vi "InputProc.vi"(7 "error in":errorcluster, 8 "output cluster":T16, 9 "SensorInputData":T17, 10 "GamepadData":T18) -> (0 "error out":errorcluster, 2 "SensorInputDataOut":T17, 3 "GamepadDataOut":T18)   [LabVIEW 2014]
uses:
  Typedefs/GamepadData.ctl
  Typedefs/SensorInputData.ctl
  <vilib>/Rock Robotics/WPI/Joystick/WPI_JoystickDevRef.ctl
  <vilib>/Rock Robotics/WPI/Joystick/WPI_JoystickDeviceEnum.ctl
  <vilib>/Rock Robotics/WPI/Potentiometer/WPI_PotentiometerDevRef.ctl
  <vilib>/Rock Robotics/SystemInterfaces/Typedef/FPGA_TypedefAnalogModule.ctl
  <vilib>/Rock Robotics/SystemInterfaces/AI/FPGA_AIChannel.ctl
  <vilib>/Rock Robotics/WPI/Encoder/WPI_EncoderDevRef.ctl
  <vilib>/Rock Robotics/SystemInterfaces/Encoder/FPGA_EncoderIdx.ctl
  <vilib>/Rock Robotics/SystemInterfaces/Counter/FPGA_CounterCtrSystemIndex.ctl
  <vilib>/Rock Robotics/WPI/Encoder/WPI_EncoderType.ctl
  <vilib>/Rock Robotics/WPI/Switch/WPI_SwitchDevRef.ctl
  <vilib>/Rock Robotics/SystemInterfaces/DIO/FPGA_DIOChannel.ctl
  <vilib>/Rock Robotics/SystemInterfaces/Typedef/FPGA_TypedefDigitalModule.ctl
  <vilib>/Rock Robotics/WPI/Gyro/WPI_GyroDevRef.ctl
  <vilib>/Rock Robotics/WPI/Compressor/WPI_CompressorDevRef.ctl
  Gensubs/Bert_or_Ernie.vi
  Typedefs/JoysticksGlobal.vi
panel:
  in  "Wench Deadzone Limit":dbl=0.05 format="%#_13g"
  in  "X360 Deadzone Limit":dbl=0.3
  in  "Bert Arm Inputs":T1={"SensorMax"=0.929, "UnitMin"=-26.5, "SensorMin"=0.502, "UnitMax"=86.8}
  in  "Ernie Arm Inputs":T1={"SensorMax"=0.837, "UnitMin"=-26.7, "SensorMin"=0.444, "UnitMax"=87.4}
  out "Claw Pot Raw":dbl
  in  "Ernie StackerClamp Inputs":T1={"SensorMax"=0.852, "UnitMin"=148.3, "SensorMin"=0.477, "UnitMax"=219.6}
  in  "Ernie Stacker Inputs":T1={"SensorMax"=0.782, "UnitMin"=0.0, "SensorMin"=0.357, "UnitMax"=21.125}
  in  "Bert StackerClamp Inputs":T1={"SensorMax"=0.42, "UnitMin"=141.5, "SensorMin"=0.064, "UnitMax"=217.6}
  out "Stacker Clamp Pot Raw":dbl format="%#_13g"
  in  "F310 Deadzone Limit":dbl=0.05
  out "Arm Pot Raw":dbl
  out "Stacker Pot Raw":dbl
  in  "Bert Stacker Inputs":T1={"SensorMax"=0.501, "UnitMin"=0.0, "SensorMin"=0.082, "UnitMax"=21.125}
  in  "ENC_CPI":dbl=0.145
  # "is now f310"
  # "ENC_CPI is encoder counts per inch"
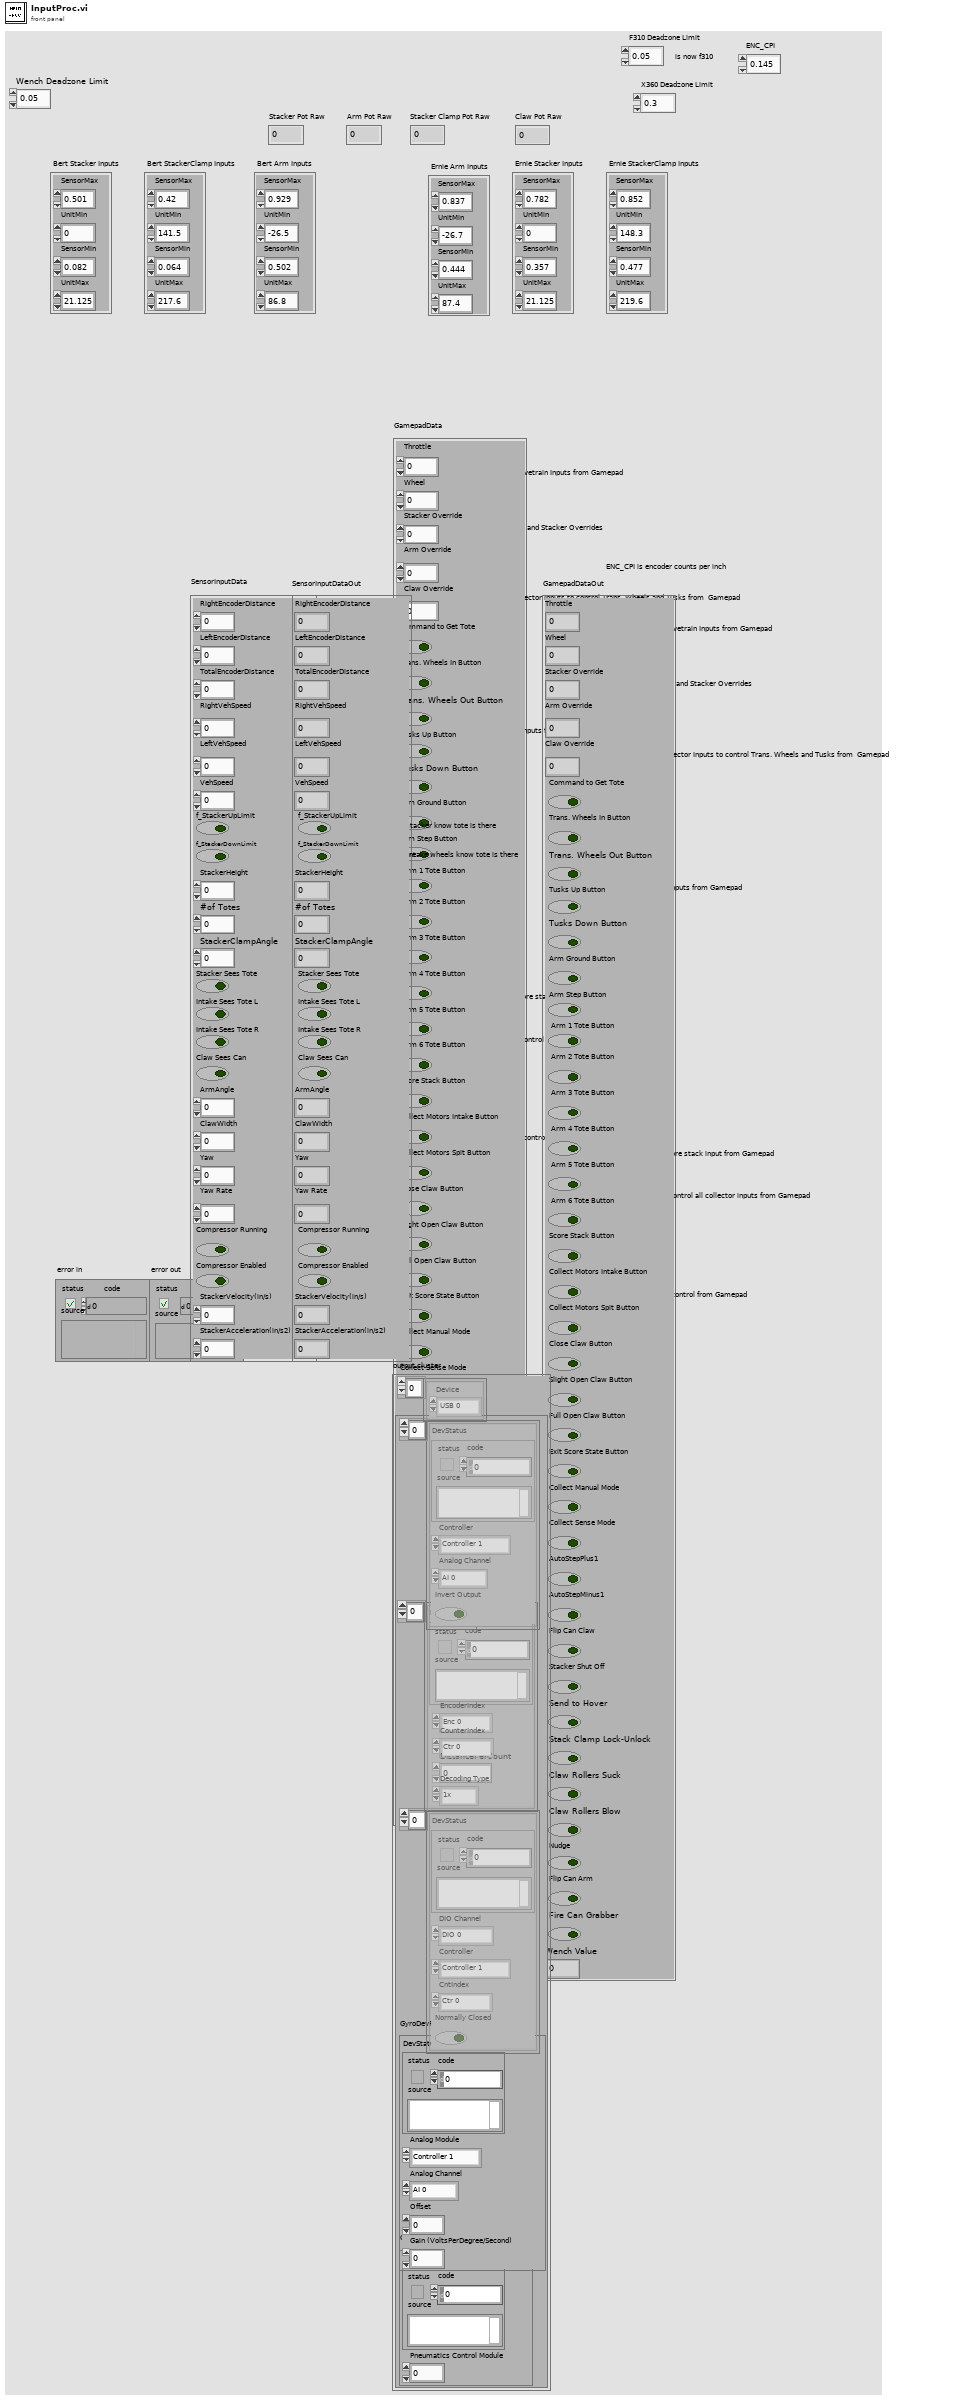
[diagram p1: front panel]
types:
  T1 = cluster{"SensorMax":dbl, "UnitMin":dbl, "SensorMin":dbl, "UnitMax":dbl}
  T2 = typedef "WPI_JoystickDevRef.ctl" = cluster{"Device":T3}
  T3 = typedef "WPI_JoystickDeviceEnum.ctl" = enum16{"USB 0", "USB 1", "USB 2", "USB 3", "USB 4", "USB 5"}
  T4 = typedef "WPI_PotentiometerDevRef.ctl" = cluster{"DevStatus":errorcluster, "Controller":T5, "Analog Channel":T6, "Invert Output":bool}
  T5 = typedef "FPGA_TypedefAnalogModule.ctl" = enum16{"Controller 1"}
  T6 = typedef "FPGA_AIChannel.ctl" = enum8{"AI 0", "AI 1", "AI 2", "AI 3", "AI MXP 0", "AI MXP 1", "AI MXP 2", "AI MXP 3", "Invalid"}
  T7 = typedef "WPI_EncoderDevRef.ctl" = cluster{"DevStatus":errorcluster, "EncoderIndex":T8, "CounterIndex":T9, "DistancePerCount":dbl, "Decoding Type":T10}
  T8 = typedef "FPGA_EncoderIdx.ctl" = enum8{"Enc 0", "Enc 1", "Enc 2", "Enc 3", "Enc 4", "Enc 5", "Enc 6", "Enc 7", "Invalid"}
  T9 = typedef "FPGA_CounterCtrSystemIndex.ctl" = enum8{"Ctr 0", "Ctr 1", "Ctr 2", "Ctr 3", "Ctr 4", "Ctr 5", "Ctr 6", "Ctr 7", "Invalid"}
  T10 = typedef "WPI_EncoderType.ctl" = enum16{"1x", "2x", "4x"}
  T11 = typedef "WPI_SwitchDevRef.ctl" = cluster{"DevStatus":errorcluster, "DIO Channel":T12, "Controller":T13, "CntIndex":T9, "Normally Closed":bool}
  T12 = typedef "FPGA_DIOChannel.ctl" = enum8{"DIO 0", "DIO 1", "DIO 2", "DIO 3", "DIO 4", "DIO 5", "DIO 6", "DIO 7", "DIO 8", "DIO 9", "DIO MXP 0", "DIO MXP 1", "DIO MXP 2", "DIO MXP 3", "DIO MXP 4", "DIO MXP 5", "DIO MXP 6", "DIO MXP 7", "DIO MXP 8", "DIO MXP 9", "DIO MXP 10", "DIO MXP 11", "DIO MXP 12", "DIO MXP 13", "DIO MXP 14", "DIO MXP 15", "Invalid"}
  T13 = typedef "FPGA_TypedefDigitalModule.ctl" = enum16{"Controller 1"}
  T14 = typedef "WPI_GyroDevRef.ctl" = cluster{"DevStatus":errorcluster, "Analog Module":T5, "Analog Channel":T6, "Offset":dbl, "Gain (VoltsPerDegree/Second)":dbl}
  T15 = typedef "WPI_CompressorDevRef.ctl" = cluster{"DevStatus":errorcluster, "Pneumatics Control Module":u8}
  T16 = cluster{T2[], cluster{T4[], T7[], T11[], "GyroDevRef":T14, "CompressorDevRef":T15}}
  T17 = typedef "SensorInputData.ctl" = cluster{"RightEncoderDistance":dbl, "LeftEncoderDistance":dbl, "TotalEncoderDistance":dbl, "RightVehSpeed":dbl, "LeftVehSpeed":dbl, "VehSpeed":dbl, "f_StackerUpLimit":bool, "f_StackerDownLimit":bool, "StackerHeight":dbl, "#of Totes":u8, "StackerClampAngle":dbl, "Stacker Sees Tote":bool, "Intake Sees Tote L":bool, "Intake Sees Tote R":bool, "Claw Sees Can":bool, "ArmAngle":dbl, "ClawWidth":dbl, "Yaw":dbl, "Yaw Rate":dbl, "Compressor Running":bool, "Compressor Enabled":bool, "StackerVelocity(in/s)":dbl, "StackerAcceleration(in/s2)":dbl}
  T18 = typedef "GamepadData.ctl" = cluster{"Throttle":dbl, "Wheel":dbl, "Stacker Override":dbl, "Arm Override ":dbl, "Claw Override":dbl, "Command to Get Tote":bool, "Trans. Wheels In Button":bool, "Trans. Wheels Out Button":bool, "Tusks Up Button":bool, "Tusks Down Button":bool, "Arm Ground Button":bool, "Arm Step Button":bool, " Arm 1 Tote Button":bool, " Arm 2 Tote Button":bool, " Arm 3 Tote Button ":bool, " Arm 4 Tote Button":bool, " Arm 5 Tote Button":bool, " Arm 6 Tote Button":bool, "Score Stack Button":bool, "Collect Motors Intake Button":bool, "Collect Motors Spit Button":bool, "Close Claw Button":bool, "Slight Open Claw Button":bool, "Full Open Claw Button ":bool, "Exit Score State Button":bool, "Collect Manual Mode ":bool, "Collect Sense Mode":bool, "AutoStepPlus1":bool, "AutoStepMinus1":bool, "Flip Can Claw":bool, "Stacker Shut Off":bool, "Send to Hover ":bool, "Stack Clamp Lock-Unlock ":bool, "Claw Rollers Suck ":bool, "Claw Rollers Blow ":bool, "Nudge":bool, "Flip Can Arm ":bool, "Fire Can Grabber":bool, "Wench Value":dbl}
  T19 = cluster{cluster{"Axes":dbl[], "Buttons":bool[], "POVs":i16[]}, cluster{"Axes":dbl[], "Buttons":bool[], "POVs":i16[]}, cluster{"Axes":dbl[], "Buttons":bool[], "POVs":i16[]}}
  T20 = cluster{"Axes":dbl[], "Buttons":bool[], "POVs":i16[]}
  T21 = cluster{T4[], T7[], T11[], "GyroDevRef":T14, "CompressorDevRef":T15}
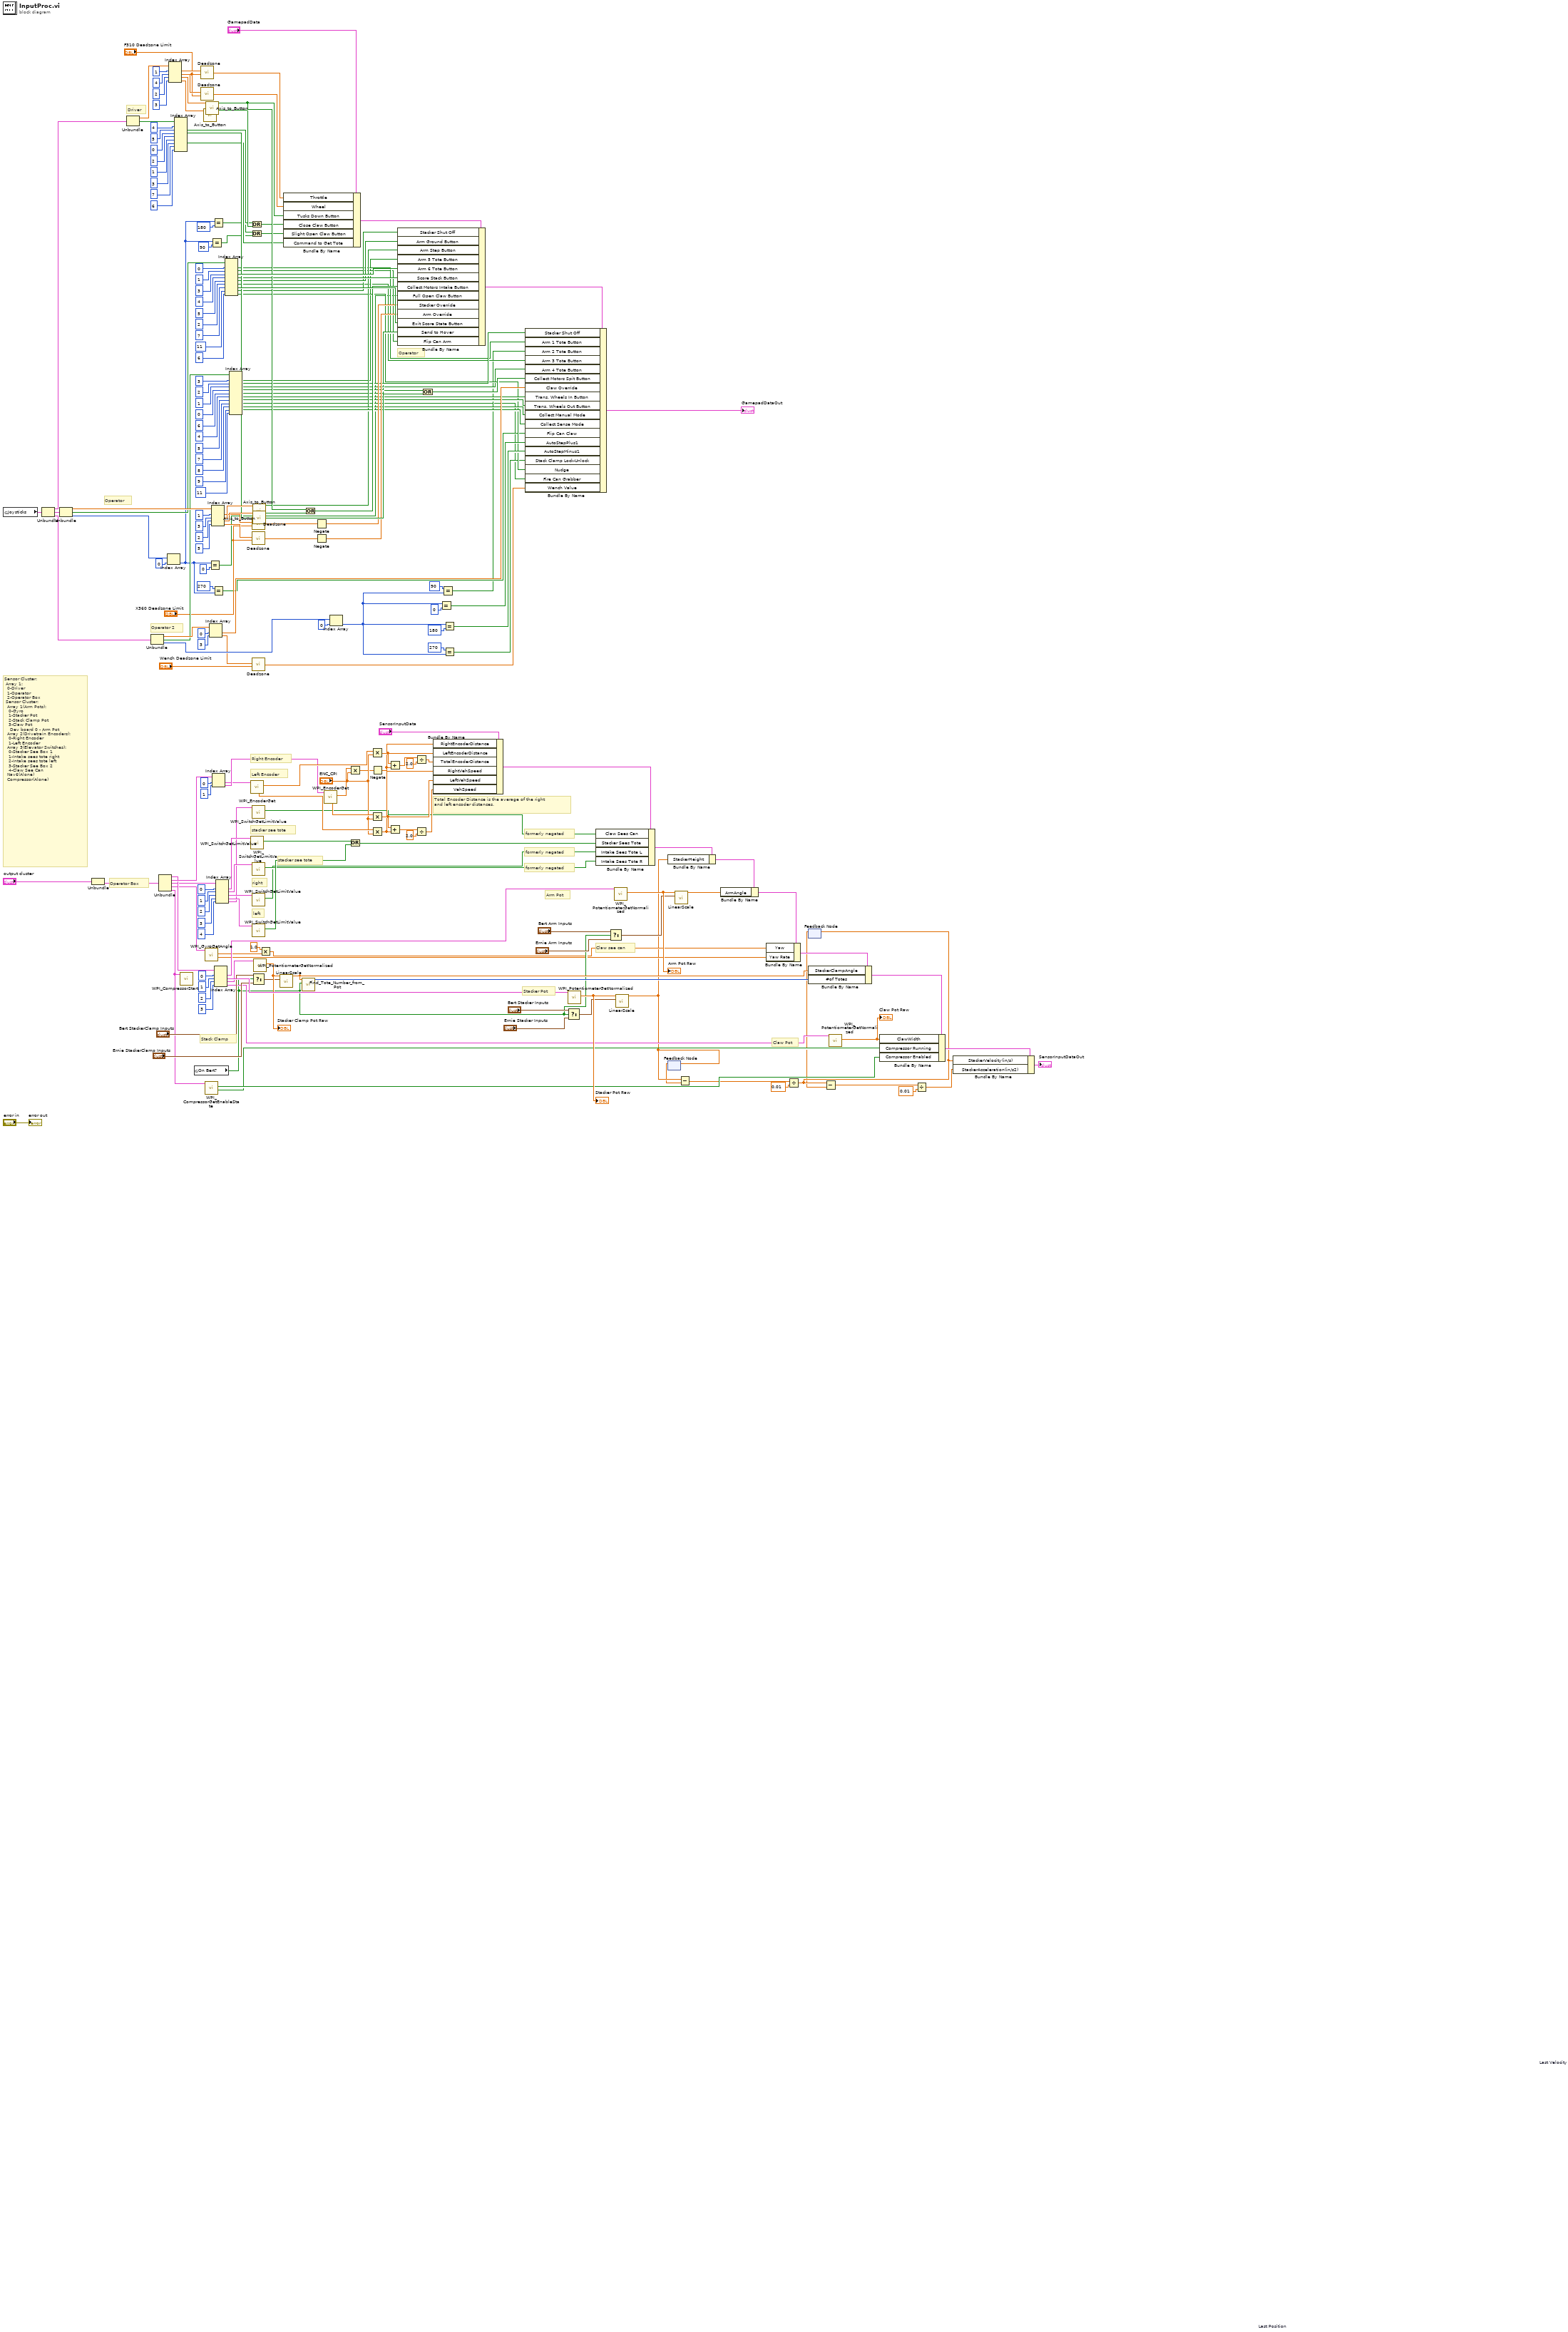
[diagram p0: block diagram]
diagram:
  # "formerly negated"
  # "right"
  # "formerly negated"
  # "formerly negated"
  # "Operator 2"
  # "Operator"
  # "Driver"
  # "Sensor Cluster:\n Array 1:\n  0-Driver\n  1-Operator\n  2-Operator Box\n Sensor Cluster:\n  Array 1(Arm Pots):\n   0-Gyro\n   1-Stacker Pot\n   2-Stack Clamp Pot\n   3-Claw Pot\n    Dev board 0 - Arm Pot\n  Array 2(Drivetrain Encoders):\n   0-Right Encoder\n   1-Left Encoder\n  Array 3(Elevator Switches):\n   0-Stacker See Box 1\n   1-Intake sees tote right\n   2-Intake sees tote left\n   3-Stacker See Box 2\n   4-Claw See Can \n  Nav6(Alone)\n  Compressor(Alone)"
  # "Claw see can"
  # "Claw Pot"
  # "stacker see tote"
  # "stacker see tote"
  # "Operator"
  # "Stack Clamp"
  # "left"
  # "Operator Box"
  # "Arm Pot"
  # "Stacker Pot"
  # "Right Encoder"
  # "Left Encoder"
  # "Total Encoder Distance is the average of the right\nand left encoder distances."
  n1 = global read "JoysticksGlobal.vi" "Joysticks"() -> (w57:T19)
  n2 = Unbundle(w57) -> (w56:T20, w50:T20, w45:T20)
  n3 = Unbundle(w50) -> ("Axes"=w53:dbl[], "Buttons"=w52:bool[], "POVs"=w51:i16[])
  n4 = Unbundle("output cluster") -> (w115:T21)  [unwired: 1 out]
  n5 = Unbundle(w56) -> ("Axes"=w55:dbl[], "Buttons"=w54:bool[])  [unwired: 1 out]
  n6 = Unbundle(w45) -> ("Axes"=w49:dbl[], "Buttons"=w48:bool[], "POVs"=w47:i16[])
  n7 = Unbundle(w115) -> (w195:T4[], w197:T7[], w190:T11[], "GyroDevRef"=w40:T14, "CompressorDevRef"=w114:T15)
  n8 = Index Array(array=w51, index=0) -> (element=w22:i16)
  n9 = Index Array(array=w55, index #1=1 ("index"), index #2=4 ("index"), index #3=2 ("index"), index #4=3 ("index")) -> (element #1=w158:dbl, element #2=w157:dbl, element #3=w179:dbl, element #4=w177:dbl)
  n10 = Index Array(array=w54, index #1=4 ("index"), index #2=5 ("index"), index #3=0 ("index"), index #4=2 ("index"), index #5=1 ("index"), index #6=3 ("index"), index #7=7 ("index"), index #8=6 ("index")) -> (element #2=w75:bool, element #3=w142:bool, element #6=w126:bool)  [unwired: 5 out]
  n11 = call <vilib>:"WPI_CompressorStart.vi"("CompressorDevRef"=w114) -> ()  [unwired: 9 in, 2 out]
  n12 = global read "Bert_or_Ernie.vi" "On Bert?"() -> (w67:bool)
  n13 = call "Deadzone.vi"("Deadzone Limit"="F310 Deadzone Limit", "Value In"=w158) -> ("Value Out"=w159:dbl)  [unwired: 4 in]
  n14 = call "Deadzone.vi"("Deadzone Limit"="F310 Deadzone Limit", "Value In"=w157) -> ("Value Out"=w160:dbl)  [unwired: 4 in]
  n15 = call "Axis_to_Button.vi"("Axis"=w177) -> ("Signal"=w89:bool)  [unwired: 10 in]
  n16 = call <vilib>:"WPI_GyroGetAngle.vi"("GyroDevRef"=w40) -> ("Angular Rate"=w38:dbl, "Angle"=w39:dbl)  [unwired: 7 in, 2 out]
  n17 = call <vilib>:"WPI_CompressorGetEnableState.vi"("CompressorDevRef"=w114) -> ("Compressor Running"=w112:bool, "Enabled"=w113:bool)  [unwired: 7 in, 2 out]
  n18 = call "Axis_to_Button.vi"("Axis"=w179) -> ("Signal"=w144:bool)  [unwired: 10 in]
  n19 = Equal?(x=w22, y=i16 0) -> (x = y?=w2:bool)
  n20 = Index Array(array=w49, index #1=0 ("index"), index #2=3 ("index")) -> (element #1=w119:dbl, element #2=w6:dbl)
  n21 = Equal?(x=w22, y=i16 90) -> (x = y?=w78:bool)
  n22 = Index Array(array=w53, index #1=1 ("index"), index #2=3 ("index"), index #3=2 ("index"), index #4=5 ("index")) -> (element #1=w84:dbl, element #2=w174:dbl, element #3=w175:dbl, element #4=w87:dbl)
  n23 = Equal?(x=w22, y=i16 180) -> (x = y?=w76:bool)
  n24 = Equal?(x=i16 270 ("y"), y=w22) -> (x = y?=w16:bool)
  n25 = Index Array(array=w197, index #1=0 ("index"), index #2=1 ("index")) -> (element #1=w189:T7, element #2=w196:T7)
  n26 = Index Array(array=w195, index #1=0 ("index"), index #2=1 ("index"), index #3=2 ("index"), index #4=3 ("index")) -> (element #1=w192:T4, element #2=w191:T4, element #3=w140:T4, element #4=w121:T4)
  n27 = Index Array(array=w190, index #1=0 ("index"), index #2=1 ("index"), index #3=2 ("index"), index #4=3 ("index"), index #5=4 ("index")) -> (element #1=w162:T11, element #2=w154:T11, element #3=w153:T11, element #4=w150:T11, element #5=w117:T11)
  n28 = Index Array(array=w52, index #1=0 ("index"), index #2=1 ("index"), index #3=3 ("index"), index #4=4 ("index"), index #5=5 ("index"), index #6=2 ("index"), index #7=7 ("index"), index #8=11 ("index"), index #9=6 ("index")) -> (element #1=w19:bool, element #2=w18:bool, element #3=w169:bool, element #4=w82:bool, element #5=w80:bool, element #6=w13:bool, element #7=w165:bool, element #8=w60:bool, element #9=w17:bool)
  n29 = Index Array(array=w48, index #1=3 ("index"), index #2=2 ("index"), index #3=1 ("index"), index #4=0 ("index"), index #5=6 ("index"), index #6=4 ("index"), index #7=5 ("index"), index #8=7 ("index"), index #9=8 ("index"), index #10=9 ("index"), index #11=11 ("index")) -> (element #1=w14:bool, element #2=w41:bool, element #3=w37:bool, element #4=w15:bool, element #5=w10:bool, element #6=w74:bool, element #7=w73:bool, element #8=w9:bool, element #9=w93:bool, element #10=w91:bool)  [unwired: 1 out]
  n30 = Or(x=w76, y=w89) -> (x .or. y?=w88:bool)
  n31 = Or(x=w75, y=w78) -> (x .or. y?=w77:bool)
  n32 = call <vilib>:"WPI_EncoderGet.vi"("EncoderDevRef"=w189) -> ("Distance"=w209:dbl, "Rate"=w106:dbl)  [unwired: 5 in, 4 out]
  n33 = call <vilib>:"WPI_SwitchGetLimitValue.vi"("SwitchDevRef"=w162) -> ("Switch Pressed"=w149:bool)  [unwired: 8 in, 2 out]
  n34 = call "Deadzone.vi"("Deadzone Limit"="X360 Deadzone Limit", "Value In"=w84) -> ("Value Out"=w83:dbl)  [unwired: 4 in]
  n35 = call "Deadzone.vi"("Deadzone Limit"="X360 Deadzone Limit", "Value In"=w87) -> ("Value Out"=w86:dbl)  [unwired: 4 in]
  n36 = call "Deadzone.vi"("Deadzone Limit"="Wench Deadzone Limit", "Value In"=w6) -> ("Value Out"=w5:dbl)  [unwired: 4 in]
  n37 = call <vilib>:"WPI_SwitchGetLimitValue.vi"("SwitchDevRef"=w154) -> ("Switch Pressed"=w4:bool)  [unwired: 8 in, 2 out]
  n38 = call <vilib>:"WPI_SwitchGetLimitValue.vi"("SwitchDevRef"=w117) -> ("Switch Pressed"=w1:bool)  [unwired: 8 in, 2 out]
  n39 = call <vilib>:"WPI_SwitchGetLimitValue.vi"("SwitchDevRef"=w153) -> ("Switch Pressed"=w3:bool)  [unwired: 8 in, 2 out]
  n40 = call <vilib>:"WPI_SwitchGetLimitValue.vi"("SwitchDevRef"=w150) -> ("Switch Pressed"=w147:bool)  [unwired: 8 in, 2 out]
  n41 = Select(t="Bert StackerClamp Inputs", s=w67, f="Ernie StackerClamp Inputs") -> (s? t:f=w134:T1)
  n42 = call "Axis_to_Button.vi"("Axis"=w174) -> ("Signal"=w81:bool)  [unwired: 10 in]
  n43 = call "Axis_to_Button.vi"("Axis"=w175) -> ("Signal"=w145:bool)  [unwired: 10 in]
  n44 = call <vilib>:"WPI_PotentiometerGetNormalized.vi"("PotDevRef"=w140) -> ("Normalized Value"=w139:dbl)  [unwired: 8 in, 2 out]
  "Stacker Clamp Pot Raw" <- w139
  n45 = Multiply(x=1.0, y=w39) -> (x*y=w59:dbl)
  n46 = call "LinearScale.vi"("RawInput"=w139, "UnitsPlease Inputs"=w134) -> ("UnitOutput"=w136:dbl)  [unwired: 13 in]
  n47 = Bundle By Name(cluster="GamepadData", "Throttle"=w159, "Wheel"=w160, "Tusks Down Button"=w144, "Close Claw Button"=w88, "Slight Open Claw Button"=w77, "Command to Get Tote"=w126) -> (w212:T18)
  n48 = call "Find_Tote_Number_from_Pot.vi"("On Bert?"=w67, "Stack Clamp Angle"=w136) -> ("Number of Totes"=w137:i8)  [unwired: 9 in]
  n49 = Or(x=w144, y=w145) -> (x .or. y?=w146:bool)
  n50 = Negate(x=w83) -> (-x=w99:dbl)
  n51 = Negate(x=w86) -> (-x=w98:dbl)
  n52 = call <vilib>:"WPI_EncoderGet.vi"("EncoderDevRef"=w196) -> ("Distance"=w208:dbl, "Rate"=w107:dbl)  [unwired: 5 in, 4 out]
  n53 = Index Array(array=w47, index=0) -> (element=w21:i16)
  n54 = Multiply(x=w208, y="ENC_CPI") -> (x*y=w43:dbl)
  n55 = Or(x=w149, y=w147) -> (x .or. y?=w148:bool)
  n56 = Multiply(x=w209, y="ENC_CPI") -> (x*y=w44:dbl)
  n57 = Multiply(x=w107, y="ENC_CPI") -> (x*y=w105:dbl)
  n58 = Multiply(x=w106, y="ENC_CPI") -> (x*y=w104:dbl)
  n59 = Negate(x=w43) -> (-x=w42:dbl)
  n60 = Add(x=w44, y=w42) -> (x+y=w206:dbl)
  n61 = Add(x=w105, y=w104) -> (x+y=w103:dbl)
  n62 = Bundle By Name(cluster=w212, "Stacker Shut Off"=w60, "Arm Ground Button"=w80, "Arm Step Button"=w81, "Arm 5 Tote Button"=w14, "Arm 6 Tote Button"=w169, "Score Stack Button"=w82, "Collect Motors Intake Button"=w146, "Full Open Claw Button"=w2, "Stacker Override"=w99, "Arm Override"=w98, "Exit Score State Button"=w165, "Send to Hover"=w37, "Flip Can Arm"=w18) -> (w183:T18)
  n63 = Divide(x=w206, y=2.0) -> (x/y=w205:dbl)
  n64 = Divide(x=w103, y=2.0) -> (x/y=w102:dbl)
  n65 = Or(x=w10, y=w142) -> (x .or. y?=w143:bool)
  n66 = Bundle By Name(cluster="SensorInputData", "RightEncoderDistance"=w42, "LeftEncoderDistance"=w44, "TotalEncoderDistance"=w205, "RightVehSpeed"=w104, "LeftVehSpeed"=w105, "VehSpeed"=w102) -> (w203:T17)
  n67 = Equal?(x=w21, y=i16 0) -> (x = y?=w63:bool)
  n68 = Equal?(x=i16 90 ("y"), y=w21) -> (x = y?=w12:bool)
  n69 = Equal?(x=w21, y=i16 180) -> (x = y?=w62:bool)
  n70 = Equal?(x=i16 270 ("y"), y=w21) -> (x = y?=w11:bool)
  n71 = Bundle By Name(cluster=w183, "Stacker Shut Off"=w41, "Arm 1 Tote Button"=w19, "Arm 2 Tote Button"=w12, "Arm 3 Tote Button"=w13, "Arm 4 Tote Button"=w15, "Collect Motors Spit Button"=w143, "Claw Override"=w119, "Trans. Wheels In Button"=w74, "Trans. Wheels Out Button"=w73, "Collect Manual Mode"=w93, "Collect Sense Mode"=w91, "Flip Can Claw"=w16, "AutoStepPlus1"=w63, "AutoStepMinus1"=w62, "Stack Clamp Lock-Unlock"=w11, "Nudge"=w17, "Fire Can Grabber"=w9, "Wench Value"=w5) -> (→"GamepadDataOut":T18)
  n72 = Select(t="Bert Stacker Inputs", s=w67, f="Ernie Stacker Inputs") -> (s? t:f=w130:T1)
  n73 = call <vilib>:"WPI_PotentiometerGetNormalized.vi"("PotDevRef"=w191) -> ("Normalized Value"=w181:dbl)  [unwired: 8 in, 2 out]
  "Stacker Pot Raw" <- w181
  n74 = Bundle By Name(cluster=w203, "Claw Sees Can"=w1, "Stacker Sees Tote"=w148, "Intake Sees Tote L"=w3, "Intake Sees Tote R"=w4) -> (w202:T17)
  n75 = Select(t="Bert Arm Inputs", s=w67, f="Ernie Arm Inputs") -> (s? t:f=w69:T1)
  n76 = call <vilib>:"WPI_PotentiometerGetNormalized.vi"("PotDevRef"=w192) -> ("Normalized Value"=w72:dbl)  [unwired: 8 in, 2 out]
  "Arm Pot Raw" <- w72
  n77 = call "LinearScale.vi"("RawInput"=w181, "UnitsPlease Inputs"=w130) -> ("UnitOutput"=w33:dbl)  [unwired: 13 in]
  n78 = Bundle By Name(cluster=w202, "StackerHeight"=w33) -> (w201:T17)
  n79 = feedback-in #1(w33) -> ()
  n80 = feedback #1 "Last Position"() -> (w32:dbl)  [unwired: 1 in]
  n81 = call "LinearScale.vi"("RawInput"=w72, "UnitsPlease Inputs"=w69) -> ("UnitOutput"=w71:dbl)  [unwired: 13 in]
  n82 = Subtract(x=w33, y=w32) -> (x-y=w30:dbl)
  n83 = Bundle By Name(cluster=w201, "ArmAngle"=w71) -> (w200:T17)
  n84 = Bundle By Name(cluster=w200, "Yaw"=w59, "Yaw Rate"=w38) -> (w138:T17)
  n85 = Divide(x=w30, y=0.01) -> (x/y=w29:dbl)
  n86 = feedback #2 "Last Velocity"() -> (w28:dbl)  [unwired: 1 in]
  n87 = feedback-in #2(w29) -> ()
  n88 = Bundle By Name(cluster=w138, "StackerClampAngle"=w136, "#of Totes"=w137) -> (w122:T17)
  n89 = Subtract(x=w29, y=w28) -> (x-y=w27:dbl)
  n90 = call <vilib>:"WPI_PotentiometerGetNormalized.vi"("PotDevRef"=w121) -> ("Normalized Value"=w116:dbl)  [unwired: 8 in, 2 out]
  "Claw Pot Raw" <- w116
  n91 = Bundle By Name(cluster=w122, "ClawWidth"=w116, "Compressor Running"=w112, "Compressor Enabled"=w113) -> (w35:T17)
  n92 = Divide(x=w27, y=0.01) -> (x/y=w25:dbl)
  n93 = Bundle By Name(cluster=w35, "StackerVelocity(in/s)"=w29, "StackerAcceleration(in/s2)"=w25) -> (→"SensorInputDataOut":T17)
  "error out" <- "error in"
